vi "GetChartParams.vi"(8 "error in (no error)":errorcluster, 10 "GraphInfoCluster":T1={"RT Display Reader Loop Time [ms]"=1000, "NI9205 Offset"={"NI9205 Offset"=[]}, "NI9205 Multiplier"={"NI9205 Multiplier"=[]}, "NI9208 Offset"={"NI9208 Offset"=[]}, "NI9208 Multiplier"={"NI9208 Multiplier"=[]}}, 11 "DisplayWaveforms":refnum<class "DisplayWaveforms.lvclass">) -> (0 "error out":errorcluster, 2 "ChartParams":T7, 3 "DisplayWaveforms out":refnum<class "DisplayWaveforms.lvclass">)   [LabVIEW 2020, in "DisplayWaveform.lvlib" / "DisplayWaveforms.lvclass"]
doc: "Get Chart Attributes to send to Chart UI"
uses:
  DisplayWaveforms.lvclass
  DisplayWaveforms.lvclass/DisplayWaveforms.ctl
  PumpMeas/TypeDefs/ChartParamsCluster.ctl
  PumpMeas/TypeDefs/NI9208multiplier.ctl
  PumpMeas/TypeDefs/NI9208offset.ctl
  PumpMeas/TypeDefs/NI9205multiplier.ctl
  PumpMeas/TypeDefs/NI9205offset.ctl
  PumpMeas/TypeDefs/RTdisplayTimedLoop_dt.ctl
  PumpMeas/TypeDefs/GraphInfoCluster.ctl
panel:
  # "For instructions on how to use the JKI State Machine Objects, examples and video tutorials, visit:\nhttp://jki.net/state-machine-objects/\n\nJKI State Machine Objects™\nhttp://jki.net/state-machine-objects/\nCopyright (C) 2005-2015, JKI <info@jki.net>\nALL RIGHTS RESERVED"
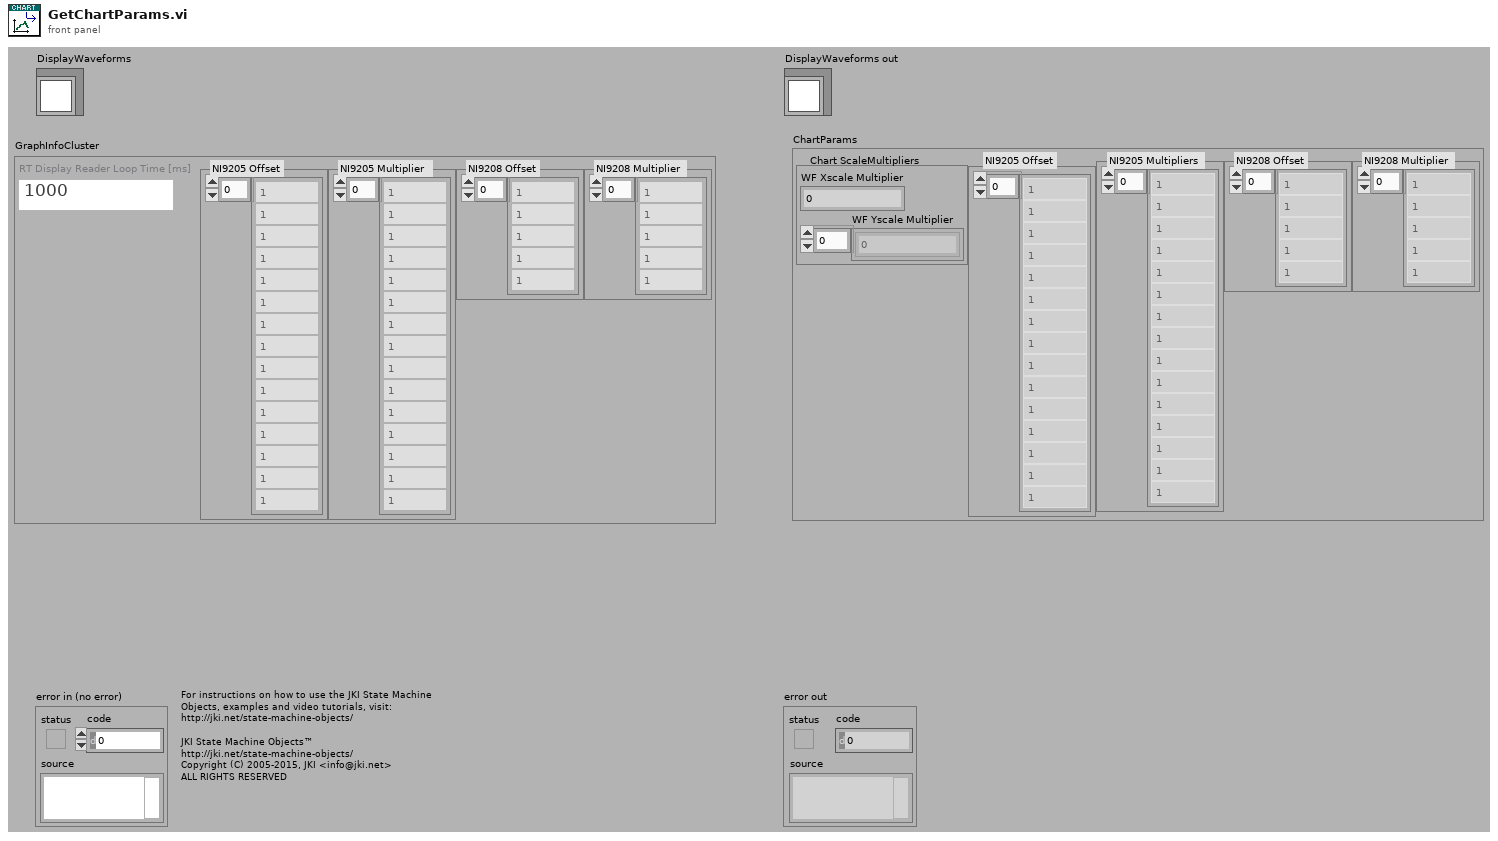
[diagram p1: front panel]
types:
  T1 = typedef "GraphInfoCluster.ctl" = cluster{"RT Display Reader Loop Time [ms]":T2, "NI9205 Offset":T3, "NI9205 Multiplier":T4, "NI9208 Offset":T5, "NI9208 Multiplier":T6}
  T2 = typedef "RTdisplayTimedLoop_dt.ctl" = i64
  T3 = typedef "NI9205offset.ctl" = cluster{"NI9205 Offset":dbl[]}
  T4 = typedef "NI9205multiplier.ctl" = cluster{"NI9205 Multiplier":dbl[]}
  T5 = typedef "NI9208offset.ctl" = cluster{"NI9208 Offset":dbl[]}
  T6 = typedef "NI9208multiplier.ctl" = cluster{"NI9208 Multiplier":dbl[]}
  T7 = typedef "ChartParamsCluster.ctl" = cluster{"Chart ScaleMultipliers":cluster{"WF Xscale Multiplier":dbl, "WF Yscale Multiplier":dbl[]}, "NI9205 Offset":T3, "NI9205 Multipliers":T4, "NI9208 Offset":T5, "NI9208 Multiplier":T6}
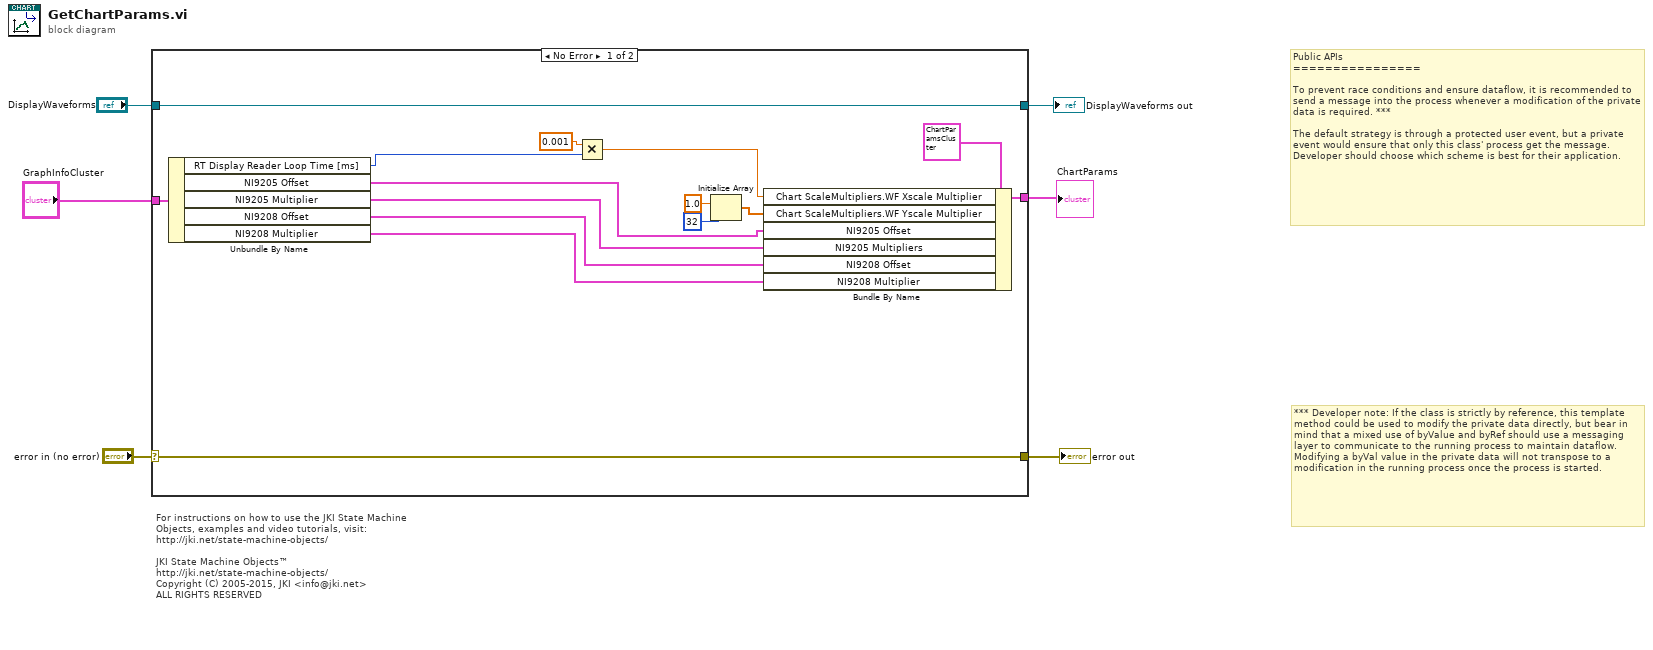
[diagram p0: block diagram]
diagram:
  # "*** Developer note: If the class is strictly by reference, this template method could be used to modify the private data directly, but bear in mind that a mixed use of byValue and byRef should use a messaging layer to communicate to the running process to maintain dataflow. Modifying a byVal value in the private data will not transpose to a modification in the running process once the process is started."
  # "Public APIs\n================\n\nTo prevent race conditions and ensure dataflow, it is recommended to send a message into the process whenever a modification of the private data is required. ***\n\nThe default strategy is through a protected user event, but a private event would ensure that only this class' process get the message. Developer should choose which scheme is best for their application."
  # "For instructions on how to use the JKI State Machine Objects, examples and video tutorials, visit:\nhttp://jki.net/state-machine-objects/\n\nJKI State Machine Objects™\nhttp://jki.net/state-machine-objects/\nCopyright (C) 2005-2015, JKI <info@jki.net>\nALL RIGHTS RESERVED"
  n1 = case shown="No Error" "error in (no error)" {
    selector: "error in (no error)" -> [w15 w22]
    tunnel: "DisplayWaveforms" -> [w21 w23]
    tunnel: [w15 w22] -> w5
    tunnel: [w21 w23] -> w4
    tunnel: "GraphInfoCluster" -> [w20 _]
    tunnel: [w19 _] -> w1
    frame No Error {
      n2 = Unbundle By Name(w20) -> ("RT Display Reader Loop Time [ms]"=w17:T2, "NI9205 Offset"=w13:T3, "NI9205 Multiplier"=w12:T4, "NI9208 Offset"=w11:T5, "NI9208 Multiplier"=w10:T6)
      n3 = Multiply(x=0.001, y=w17) -> (x*y=w14:dbl)
      n4 = Initialize Array(1.0 ("element"), 32 ("dimension size")) -> (w7:dbl[])
      n5 = Bundle By Name(cluster=T7 {"Chart ScaleMultipliers"={"WF Xscale Multiplier"=0.0, "WF Yscale Multiplier"=[]}, "NI9205 Offset"={"NI9205 Offset"=[]}, "NI9205 Multipliers"={"NI9205 Multiplier"=[]}, "NI9208 Offset"={"NI9208 Offset"=[]}, "NI9208 Multiplier"={"NI9208 Multiplier"=[]}} ("ChartParams"), "Chart ScaleMultipliers.WF Xscale Multiplier"=w14, "Chart ScaleMultipliers.WF Yscale Multiplier"=w7, "NI9205 Offset"=w13, "NI9205 Multipliers"=w12, "NI9208 Offset"=w11, "NI9208 Multiplier"=w10) -> (w19:T7)
    }
    frame Error {
    }
  }
  "error out" <- w5
  "DisplayWaveforms out" <- w4
  "ChartParams" <- w1
